vi "VNS Engine For Local Searcher Module.vi"(0 "Best Chromosome In":u16[](array[numeric])=[1, 7, 8, 14, 6, 15, 11, 12, 3, 9, 5, 10, 4, 13, 0, 2], 1 "Processing Times":u16[][](array[numeric]), 5 "Number of Machines":i32, 7 "Number of Jobs":i32, 9 "Max Iteration Count":i32=1, 11 "error in (no error)":errorcluster, 12 "Due Dates":u16[](array[numeric])) -> (4 "VNS Result":u16[](array[numeric]), 8 "Tardiness(FIFO Engine)":u16, 15 "error out":errorcluster)   [LabVIEW 2013]
uses:
  GA/SubVIS/Remove Duplicates In Array.vi
  Classes/Scheduler_Class/Prins FIFO Scheduler Methods and Controls/Prins FIFO Scheduler.vi
  Classes/Scheduler_Class/Prins FIFO Scheduler Methods and Controls/Methods/Calculate Final Completion Times of Jobs.vi
  Classes/Scheduler_Class/Prins FIFO Scheduler Methods and Controls/Methods/Reorder Schedule(Prins FIFO) based on Start Times.vi
  GA/SubVIS/Calcualte General Tardiness.vi
  Classes/Scheduler_Class/Prins FIFO Scheduler Methods and Controls/Methods/UpdateMachineGaps.vi
  Classes/Scheduler_Class/Prins FIFO Scheduler Methods and Controls/Methods/UpdateJobGaps.vi
  Classes/Scheduler_Class/Prins FIFO Scheduler Methods and Controls/Methods/Find Intersecting Gaps.vi
  Classes/Scheduler_Class/Prins FIFO Scheduler Methods and Controls/Methods/Transform to Plain Job and Machine Gaps Array.vi
  Classes/Scheduler.lvclass
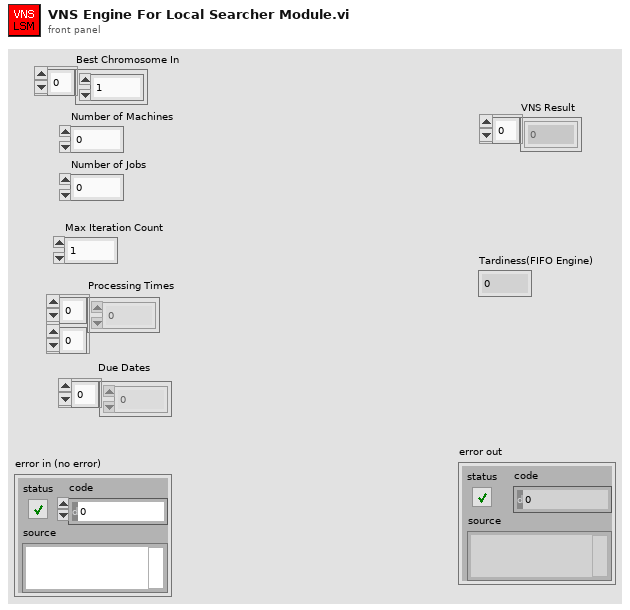
[diagram p1: front panel]
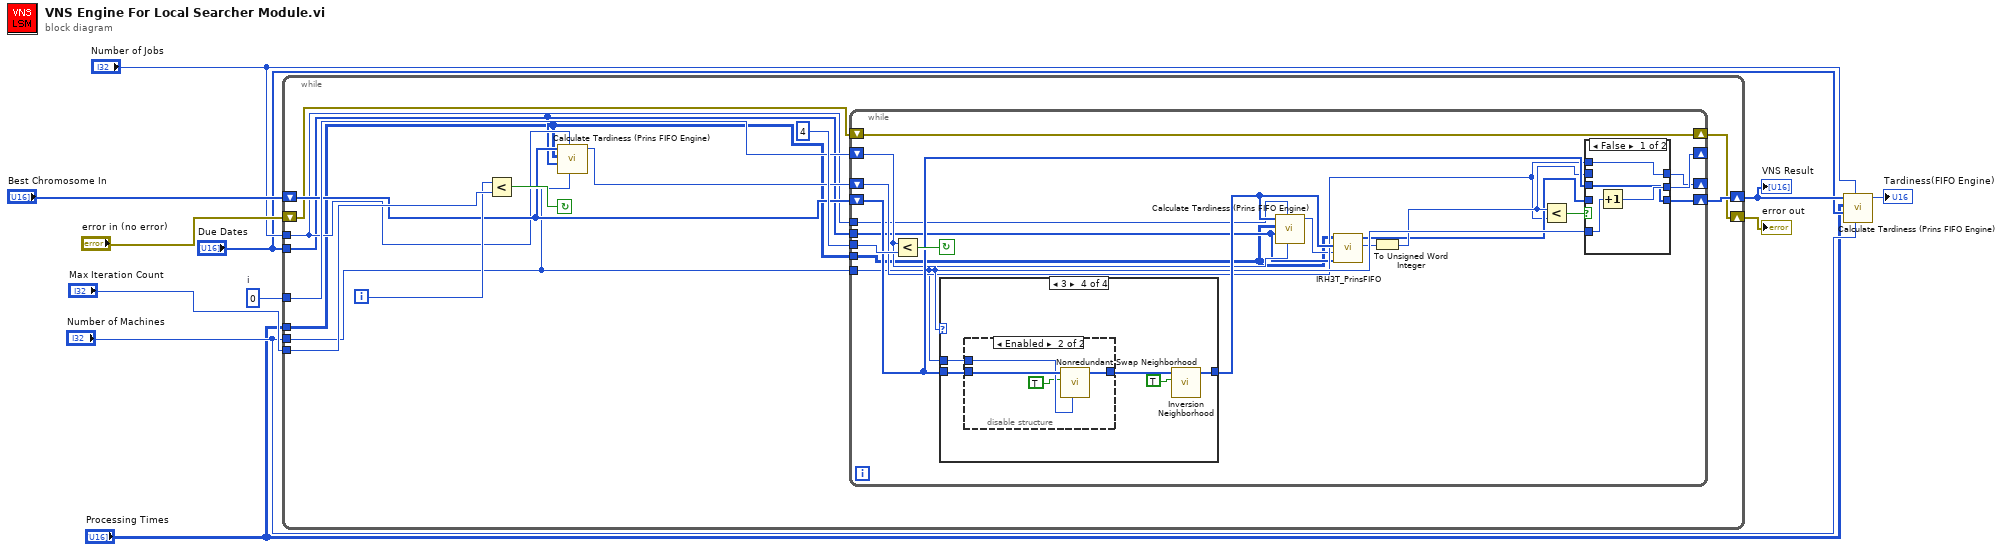
[diagram p0: block diagram]
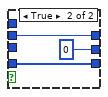
[diagram p2: hidden frame]
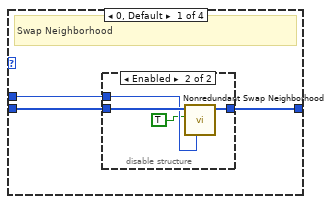
[diagram p3: hidden frame]
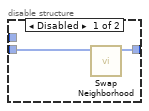
[diagram p4: hidden frame]
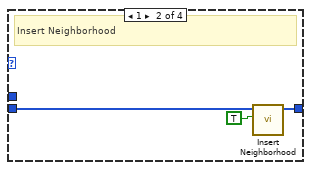
[diagram p5: hidden frame]
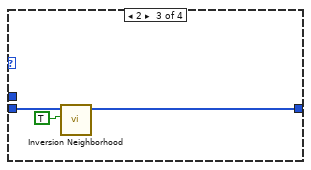
[diagram p6: hidden frame]
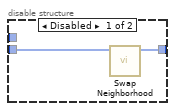
[diagram p7: hidden frame]
diagram:
  w10 = 0  # i
  n1 = while {
    tunnel: "Max Iteration Count" -> [w25]
    tunnel: w10 -> [w22]
    shift-right: [w20] -> w9
    shift-left: "Best Chromosome In" -> [w18]
    shift-right: [w19] -> w1
    shift-left: "error in (no error)" -> [w15]
    tunnel: "Number of Machines" -> [w16]
    tunnel: "Number of Jobs" -> [w14]
    tunnel: "Due Dates" -> [w13]
    tunnel: "Processing Times" -> [w12]
    i -> [w21]
    stop <- w24 continue-if-true
    n2 = Less?(x=w21, y=w25) -> (x < y?=w24:bool)
    n3 = call "Calculate Tardiness (Prins FIFO Engine).vi"("Number of Machines"=w16, "Number of Jobs"=w14, "Due Dates"=w13, "Processing Times"=w12, "Schedule In"=w18) -> ("Tardiness(Prins FIFO Engine)"=w17:u16)  [unwired: 5 in, 1 out]
    n4 = while {
      tunnel: 4 -> [w41]
      shift-right: [w40] -> _
      shift-left: w22 -> [w37]
      shift-right: [w39] -> w20
      shift-left: w18 -> [w38]
      shift-right: [w26] -> w19
      shift-left: w15 -> [w26]
      shift-right: [w35] -> _
      shift-left: w17 -> [w33]
      tunnel: w16 -> [w30]
      tunnel: w14 -> [w29]
      tunnel: w13 -> [w28]
      tunnel: w12 -> [w27]
      stop <- w44 continue-if-true
      n5 = Less?(x=w37, y=w41) -> (x < y?=w44:bool)
      n6 = case shown="3" w37 {
        tunnel: w38 -> [w54 w63 w66 w71]
        tunnel: [w53 w62 w65 w69] -> w43
        tunnel: w30 -> [w52 _ _ w68]
        frame 0, Default {
          # "Swap Neighborhood"
          n7 = disable-structure shown="Enabled" {
            disable-tunnel: w54 -> [w56 w60]
            disable-tunnel: [w55 w59] -> w53
            disable-tunnel: w52 -> [_ w58]
            frame Disabled {
              n8 = call "Swap Neighborhood.vi"("Schedule In"=w56) -> ("Schedule Out"=w55:u16[])  [unwired: 10 in]
            }
            frame Enabled {
              n9 = call "Nonredundant Swap Neighborhood.vi"("Number of Machines"=w58, "Generate Random indices?"=TRUE, "Schedule in"=w60) -> ("Schedule out"=w59:u16[])  [unwired: 8 in]
            }
          }
        }
        frame 1 {
          # "Insert Neighborhood"
          n10 = call "Insert Neighborhood.vi"("Generate Random Indices?"=TRUE, "C'"=w63) -> ("Chromosome Out"=w62:u16[])  [unwired: 9 in]
        }
        frame 2 {
          n11 = call "Inversion Neighborhood.vi"("Generate Random Indices?"=TRUE, "Schedule in"=w66) -> ("Schedule out"=w65:u16[])  [unwired: 9 in]
        }
        frame 3 {
          n12 = disable-structure shown="Enabled" {
            disable-tunnel: w71 -> [w73 w77]
            disable-tunnel: [w72 w76] -> w70
            disable-tunnel: w68 -> [_ w75]
            frame Disabled {
              n13 = call "Swap Neighborhood.vi"("Schedule In"=w73) -> ("Schedule Out"=w72:u16[])  [unwired: 10 in]
            }
            frame Enabled {
              n14 = call "Nonredundant Swap Neighborhood.vi"("Number of Machines"=w75, "Generate Random indices?"=TRUE, "Schedule in"=w77) -> ("Schedule out"=w76:u16[])  [unwired: 8 in]
            }
          }
          n15 = call "Inversion Neighborhood.vi"("Generate Random Indices?"=TRUE, "Schedule in"=w70) -> ("Schedule out"=w69:u16[])  [unwired: 9 in]
        }
      }
      n16 = call "Calculate Tardiness (Prins FIFO Engine).vi"("Number of Machines"=w30, "Number of Jobs"=w29, "Due Dates"=w28, "Processing Times"=w27, "Schedule In"=w43) -> ("Tardiness(Prins FIFO Engine)"=w32:u16)  [unwired: 5 in, 1 out]
      n17 = call "IRH3T_PrinsFIFO.vi"("Due Dates"=w28, "Initial Tardiness"=w32, "Schedule 2B Improved"=w43, "Proocessing Times  (Machines x Jobs)"=w27) -> ("Total Tardiness"=w31:u16, "IRH3T (Reordered) Schedule Out"=w34:u16[])  [unwired: 5 in, 1 out]
      n18 = To Unsigned Word Integer(number=w31) -> (unsigned 16bit integer=w36:u16)
      n19 = Less?(x=w36, y=w33) -> (x < y?=w42:bool)
      n20 = case shown="False" w42 {
        tunnel: w37 -> [w47 _]
        tunnel: w34 -> [_ w50]
        tunnel: [w48 0] -> w40
        tunnel: [w46 w50] -> w39
        tunnel: w38 -> [w46 _]
        tunnel: w36 -> [_ w49]
        tunnel: [w45 w49] -> w35
        tunnel: w33 -> [w45 _]
        frame False {
          n21 = Increment(x=w47) -> (x+1=w48:i32)
        }
        frame True {
        }
      }
    }
  }
  "VNS Result" <- w9
  "error out" <- w1
  n22 = call "Calculate Tardiness (Prins FIFO Engine).vi"("Number of Machines"="Number of Machines", "Number of Jobs"="Number of Jobs", "Due Dates"="Due Dates", "Processing Times"="Processing Times", "Schedule In"=w9) -> ("Tardiness(Prins FIFO Engine)"=→"Tardiness(FIFO Engine)":u16)  [unwired: 5 in, 1 out]
